vi "FF_circle.vi"   [LabVIEW 2013]
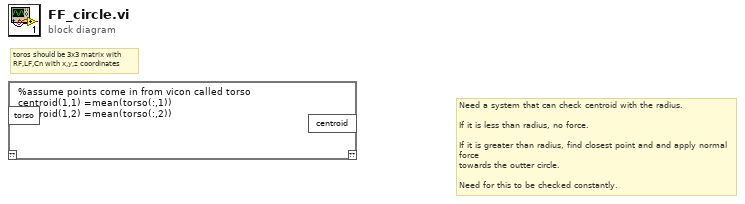
[diagram p0: block diagram]
diagram:
  # "Need a system that can check centroid with the radius.\n\nIf it is less than radius, no force.\n\nIf it is greater than radius, find closest point and and apply normal force\ntowards the outter circle.\n\nNeed for this to be checked constantly."
  # "toros should be 3x3 matrix with \nRF,LF,Cn with x,y,z coordinates"
  n1 = mathscript code="%assume points come in from vicon called torso\ncentroid(1,1) =mean(torso(:,1))\ncentroid(1,2) =mean(torso(:,2))"() -> ()  [unwired: 2 in, 2 out]
